vi "run.get_from_number.vi"(8 "error in":errorcluster, 10 "Run Number":i32, 11 "Nominal Client in":refnum<class "Nominal Client.lvclass">) -> (0 "error out":errorcluster, 2 "Run":refnum<class "Run.lvclass">, 3 "Nominal Client out":refnum<class "Nominal Client.lvclass">, 4 "Response body":string)   [LabVIEW 2020, in "Nominal Client.lvclass"]
doc: "Fetches a run based on the run number, rather than RID."
uses:
  Nominal Client.lvclass
  Run/Run.lvclass
  Nominal Client.lvclass/Nominal Client.ctl
  nominal types/workspace/workspace.lvclass/workspace.ctl
  49411445-db77-4211-b7bb-06afe579b778.vi
  workspace.get.vi
  <vilib>/JDP Science/JSONtext/Merge into Object.vi
  workspace.add_to_payload.vi/88650e10-de3e-481c-85db-71cb0fdf4485.vi
  nominal types/workspace/rid.get.vi
  <vilib>/JDP Science/JSONtext/Variant to JSON Text.vi
  <vilib>/JDP Science/JSONtext/Get all Object Items.vi
  <vilib>/JDP Science/JSONtext/Set Multiple Object Items.vi
  <vilib>/JDP Science/JSONtext/LVClass Serializer/JSONtext LVClass Serializer.lvclass
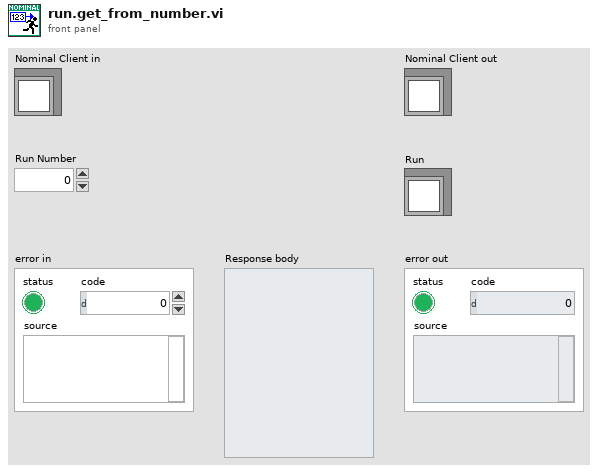
[diagram p1: front panel]
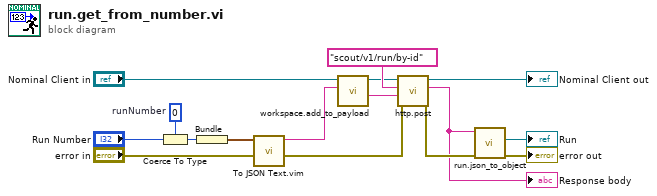
[diagram p0: block diagram]
diagram:
  w12 = 0  # runNumber
  n1 = Coerce To Type(0:"Run Number", 1:w12) -> (2:w9:i32)
  n2 = Bundle("runNumber"=w9) -> (w10:cluster{"runNumber":i32})  [unwired: 1 in]
  n3 = call "To JSON Text.vim"("error in (no error)"="error in", "Anything"=w10) -> ("error out"=w13:errorcluster, "<JSON>"=w2:string)  [unwired: 8 in]
  n4 = call "workspace.add_to_payload.vi"("JSON payload in"=w2, "Nominal Client in"="Nominal Client in") -> ("JSON payload out"=w1:string, "Nominal Client out"=w3:refnum<class "Nominal Client.lvclass">)  [unwired: 7 in, 1 out]
  n5 = call "http.post.vi"("error in"=w13, "Request body"=w1, "Path"="scout/v1/run/by-id", "Nominal Client in"=w3) -> ("error out"=w6:errorcluster, "Response"=w5:string, "Nominal Client out"=→"Nominal Client out":refnum<class "Nominal Client.lvclass">)  [unwired: 4 in, 1 out]
  "Response body" <- w5
  n6 = call "run.json_to_object.vi"("error in"=w6, "JSON"=w5) -> ("error out"=→"error out":errorcluster, "Run"=→"Run":refnum<class "Run.lvclass">)  [unwired: 8 in]
